vi "Event handler-Laser power value change.vi"(11 "Laser Power knob.NewVal":T1 caption="NewVal" max=1000 step=5 scale=0.0..100.0) -> ()   [LabVIEW 2013]
uses:
  Typedefs/Laser control knob.ctl
  Global Variables/gl_UI Ctrl Refs.vi
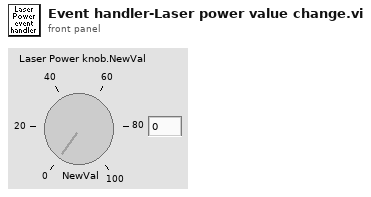
[diagram p1: front panel]
types:
  T1 = typedef "Laser control knob.ctl" = u16
  T2 = typedef "UI ctrl refs cluster.ctl" = cluster{"Top level VI path":path, "Top level VI ref":refnum<vi>, "User menu ref":refnum<k9>, "Sub Panel control":refnum<vi>, "Imaging Param Tab":refnum<vi>, "Occurrence-Start drivers":refnum<k4>, "Occurrence-Speed logging initialised":refnum<k4>, "Occurrence-XYZ stage initialised":refnum<k4>, "Exit button":refnum<vi>, "Status ind":refnum<vi>, "Return to Origin":refnum<vi>, "Speed Logging":refnum<vi>, "Time Lapse":refnum<vi>, "Live Imaging":refnum<vi>, "AOL Z Stack":refnum<vi>, "Motor Z Stack":refnum<vi>, "Funct Acq button":refnum<vi>, "Hard Shutter":refnum<vi>, "Virtual Shutter":refnum<vi>, "Laser Power":refnum<vi>, "AOL Mode":refnum<vi>, "Frame Size":refnum<vi>, "Field of View":refnum<vi>, "Dwell Time":refnum<vi>, "Zoom":refnum<vi>, "AOL Z":refnum<vi>, "Objective":refnum<vi>, "Axis":refnum<vi>, "Paths & Names":refnum<vi>, "Experiment folder path (ind.)":refnum<vi>, "Last State (Ind.)":refnum<vi>, "Laser wavelength ind (nm)":refnum<vi>, "Averages":refnum<vi>, "Angle (degrees)":refnum<vi>, "X centre":refnum<vi>, "Y centre":refnum<vi>, "Plane Mode":refnum<vi>, "# Planes":refnum<vi>, "Z Start":refnum<vi>, "Z Stop":refnum<vi>, "Z Step":refnum<vi>, "PMT 1":refnum<vi>, "PMT 2":refnum<vi>, "Stage XYZ Position":refnum<vi>, "Pockels@Z Start":refnum<vi>, "Pockels@Z Stop":refnum<vi>, "Obtain Z Start":refnum<vi>, "Obtain Z Stop":refnum<vi>, "Live stim.trig.period":refnum<vi>, "Live stim.trig.enable":refnum<vi>, "Funct. Acq. Pockels Modulation":refnum<vi>, "Enable Video Recording":refnum<vi>, "Video Record-Live Imaging":refnum<vi>, "Video Record-Funct acq":refnum<vi>, "AOL Z-stack Chirps Ready (ind)":refnum<vi>, "Center freq ind (nm)":refnum<vi>, "Logging queue (ind)":refnum<vi>, "Back aperture power (ind.)":refnum<vi>, "Power after objective (ind.)":refnum<vi>, "Switch user":refnum<vi>}
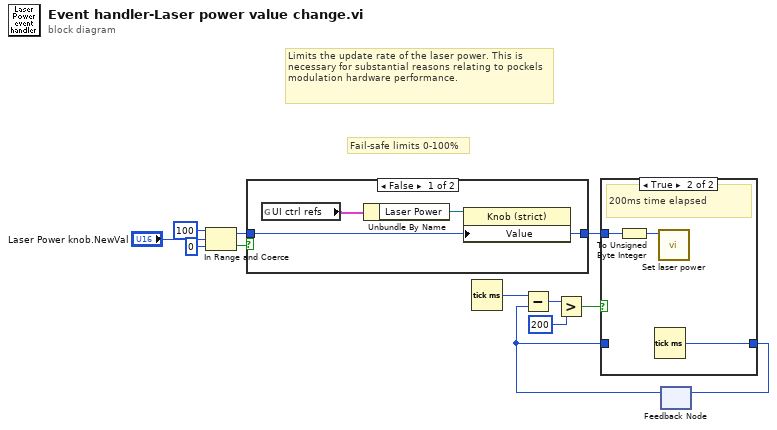
[diagram p0: block diagram]
diagram:
  # "Fail-safe limits 0-100%"
  # "Limits the update rate of the laser power. This is necessary for substantial reasons relating to pockels modulation hardware performance."
  n1 = In Range and Coerce(upper limit=T1 100, x="Laser Power knob.NewVal", lower limit=T1 0) -> (coerced(x)=w11:T1, In Range?=w12:bool)
  n2 = case shown="False" w12 {
    tunnel: w11 -> [w15 w16]
    tunnel: [w15 w16] -> w2
    frame False {
      n3 = global read "gl_UI Ctrl Refs.vi" "UI ctrl refs"() -> (w13:T2)
      n4 = Unbundle By Name(w13) -> ("Laser Power"=w14:refnum<vi>)
      n5 = property on="Property Node" class="Knob (strict)"(reference=w14, "Value"=w15) -> ()  [unwired: 1 in, 2 out]
    }
    frame True {
    }
  }
  n6 = Tick Count (ms)() -> (millisecond timer value=w3:u32)
  n7 = feedback #1() -> (w7:u32)  [unwired: 1 in]
  n8 = Subtract(x=w3, y=w7) -> (x-y=w4:u32)
  n9 = Greater?(x=w4, y=u32 200) -> (0:w6:bool)
  n10 = case shown="True" w6 {
    tunnel: [w17 w20] -> w1
    tunnel: w7 -> [w17 _]
    tunnel: w2 -> [_ w19]
    frame False {
      # "Counting towards 200ms"
    }
    frame True {
      # "200ms time elapsed"
      n11 = To Unsigned Byte Integer(number=w19) -> (unsigned 8bit integer=w18:u8)
      n12 = Tick Count (ms)() -> (millisecond timer value=w20:u32)
      n13 = call "Set laser power.vi"("Laser power %"=w18) -> ()  [unwired: 10 in, 1 out]
    }
  }
  n14 = feedback-in #1(w1) -> ()
